vi "IMU Read.vi"(6 "Configuration":T2={"Accelerometer Bias"={"X (m/s)"=0.0, "Y (m/s)"=0.0, "Z (m/s)"=0.0}, "Gyroscope Bias"={"X (m/s)"=0.0, "Y (m/s)"=0.0, "Z (m/s)"=0.0}, "Steering Motor Gear Ratio"=0.0, "Steering Pully Gear Ratio"=0.0, "Steering Encoder CPR"=0.0, "Steering Motor Max RPM"=4000.0, "Wheelbase (m)"=1.12, "Fork Angle (rad)"=1.3, "Balancing Controller"={"Kp (/s)"=0.0, "Kd (1)"=0.0}, "Max Allowed Steering Angle (rad)"=0.7, "Task Periods"={"Emergency Stop (us)"=0, "IMU (us)"=0, "Steering Motor Encoder (us)"=0, "State Estimator (us)"=0, "Balancing Controller (us)"=0, "GNSS (us)"=0, "Logging (us)"=0, "Drive Motor (us)"=0, "Visualization (us)"=50000}, "Drive Motor Gear Ratio"=0.7, "lr"=0.0, "lf"=0.0, "lambda"=0.0, "k1"=0.0, "k2"=0.0, "e1_max"=0.0, "Ad_t"=0.0, "Bd_t"=0.0, "C_t"=0.0, "D_t"=0.0, "Wheel radius"=0.311}, 8 "Measurement In":refnum<data-value>, 9 "Flag IMU":dbl, 10 "IMU Handle":T3={"I2C address"=107}, 11 "Error In":errorcluster) -> (0 "Measurement Out":refnum<data-value>, 1 "IMU Data":T1, 3 "Error Out":errorcluster)   [LabVIEW 2021]
uses:
  IMU Handle.ctl
  Configuration/Configuration.ctl
  IMU Data.ctl
  State Estimator/Measurements.ctl
  Steering Motor Encoder/Steering Motor Encoder Data.ctl
  GNSS/GNSS Data.ctl
  <vilib>/myRIO/Instrument Drivers/Onboard IO/I2C/typedefs/I2C User Configuration.ctl
  <vilib>/myRIO/Instrument Drivers/Onboard IO/I2C/typedefs/I2C Transfer Rate.ctl
  <vilib>/myRIO/Instrument Drivers/Onboard IO/I2C/typedefs/I2C Reference.ctl
  <vilib>/myRIO/Common/Instrument Driver Framework/Utilities/typedefs/myRIO Generic Hardware Reference.ctl
  <vilib>/myRIO/Common/Instrument Driver Framework/Utilities/typedefs/Hardware Version Enum.ctl
  <vilib>/myRIO/Common/Instrument Driver Framework/Utilities/typedefs/myRIO v1.0 Reference.ctl
  <vilib>/myRIO/Common/Instrument Driver Framework/Utilities/typedefs/Generic FPGA Reference.ctl
  <vilib>/myRIO/Common/Instrument Driver Framework/myRIO v1.0/I2C/typedefs/I2C Channels Enum.ctl
  <vilib>/myRIO/Instrument Drivers/Onboard IO/I2C/typedefs/I2C Configuration.ctl
  <vilib>/userDefined/High Color/nirio_resource_hc.ctl
  <vilib>/myRIO/Common/Instrument Driver Framework/Utilities/vis/Is FPGA Ref Available.vi
  <vilib>/myRIO/Common/Instrument Driver Framework/myRIO v1.0/I2C/vis/myRIO v1.1 Open I2C.vi
  <vilib>/myRIO/Instrument Drivers/Onboard IO/I2C/vis/Configure.vi
  <vilib>/myRIO/Instrument Drivers/Onboard IO/I2C/vis/Write Read.vi
  <vilib>/myRIO/Common/Instrument Driver Framework/Utilities/vis/Validate Channels.vi
  <vilib>/myRIO/Common/Instrument Driver Framework/myRIO v1.0/I2C/vis/myRIO v1.0 Reserve I2C.vi
  <vilib>/myRIO/Common/Instrument Driver Framework/myRIO v1.0/I2C/vis/myRIO v1.0 Build MUX Configuration I2C.vi
  <vilib>/myRIO/Common/Instrument Driver Framework/myRIO v1.0/Resource Manager/vis/myRIO v1.0 Reserve Channel List.vi
  <vilib>/myRIO/Common/Instrument Driver Framework/myRIO v1.0/Resource Manager/vis/myRIO v1.0 Create Configuration List.vi
  <vilib>/myRIO/Common/Instrument Driver Framework/myRIO v1.0/Resource Manager/vis/myRIO v1.0 Reserve Channel.vi
  <vilib>/myRIO/Common/Instrument Driver Framework/myRIO v1.0/Resource Manager/vis/myRIO v1.0 Unreserve Channel.vi
  <vilib>/myRIO/Common/Instrument Driver Framework/myRIO v1.0/Resource Manager/vis/myRIO v1.0 Build Mutex Name.vi
  <vilib>/Utility/VariantDataType/GetNumericInfo.vi
  <vilib>/Utility/error.llb/Error Cluster From Error Code.vi
  <vilib>/myRIO/Common/Instrument Driver Framework/myRIO v1.0/myRIO v1.1 Open.vi
  <vilib>/myRIO/Common/Instrument Driver Framework/Utilities/vis/IO Manager.vi
  <vilib>/myRIO/Common/Instrument Driver Framework/Utilities/vis/Configuration Manager.vi
  <vilib>/myRIO/Common/Instrument Driver Framework/myRIO v1.0/Resource Manager/vis/myRIO v1.0 Configure IO.vi
  <vilib>/myRIO/Common/Instrument Driver Framework/myRIO v1.0/myRIO v1.0 Close.vi
  <vilib>/myRIO/Common/Instrument Driver Framework/myRIO v1.0/I2C/vis/myRIO v1.0 Configure I2C.vi
  <vilib>/myRIO/Common/Instrument Driver Framework/myRIO v1.0/I2C/vis/myRIO v1.0 Write I2C.vi
  <vilib>/myRIO/Common/Instrument Driver Framework/myRIO v1.0/I2C/vis/myRIO v1.0 Read I2C.vi
  <vilib>/myRIO/Express VI/Onboard IO/I2C/I2C Express VI.xnode
  <vilib>/myRIO/Instrument Drivers/Onboard IO/I2C/vis/myRIO I2C Open.xnode
  <vilib>/myRIO/Instrument Drivers/Onboard IO/I2C/I2C.lvlib
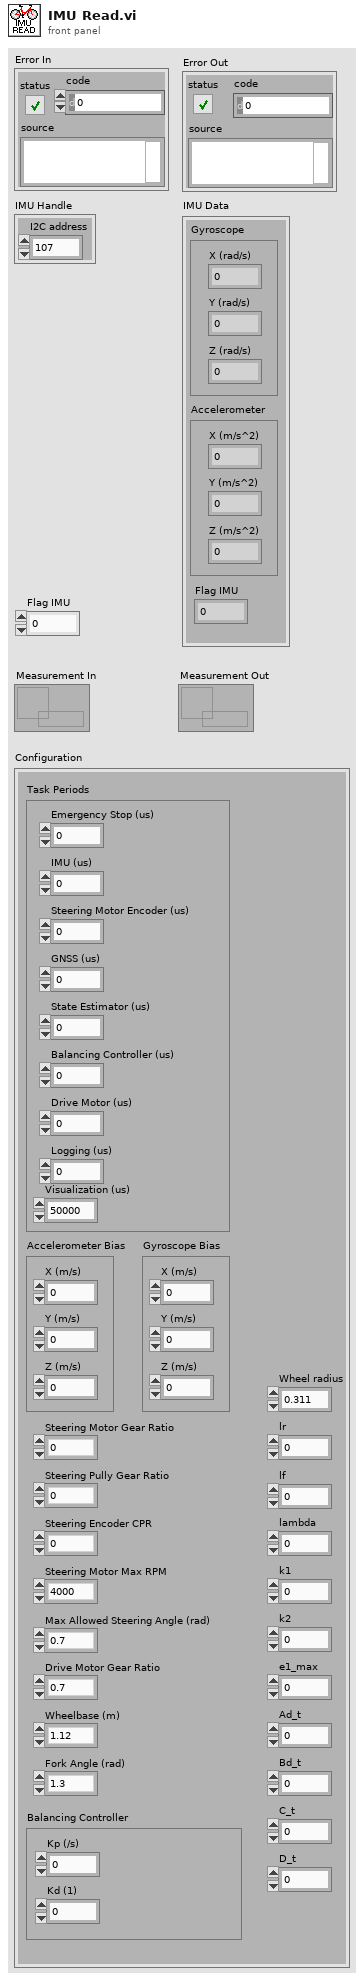
[diagram p1: front panel]
types:
  T1 = typedef "IMU Data.ctl" = cluster{"Gyroscope":cluster{"X (rad/s)":dbl, "Y (rad/s)":dbl, "Z (rad/s)":dbl}, "Accelerometer":cluster{"X (m/s^2)":dbl, "Y (m/s^2)":dbl, "Z (m/s^2)":dbl}, "Flag IMU":dbl}
  T2 = typedef "Configuration.ctl" = cluster{"Accelerometer Bias":cluster{"X (m/s)":dbl, "Y (m/s)":dbl, "Z (m/s)":dbl}, "Gyroscope Bias":cluster{"X (m/s)":dbl, "Y (m/s)":dbl, "Z (m/s)":dbl}, "Steering Motor Gear Ratio":dbl, "Steering Pully Gear Ratio":dbl, "Steering Encoder CPR":dbl, "Steering Motor Max RPM":dbl, "Wheelbase (m)":dbl, "Fork Angle (rad)":dbl, "Balancing Controller":cluster{"Kp (/s)":dbl, "Kd (1)":dbl}, "Max Allowed Steering Angle (rad)":dbl, "Task Periods":cluster{"Emergency Stop (us)":i64, "IMU (us)":i64, "Steering Motor Encoder (us)":i64, "State Estimator (us)":i64, "Balancing Controller (us)":i64, "GNSS (us)":i64, "Logging (us)":i64, "Drive Motor (us)":i64, "Visualization (us)":i64}, "Drive Motor Gear Ratio":dbl, "lr":dbl, "lf":dbl, "lambda":dbl, "k1":dbl, "k2":dbl, "e1_max":dbl, "Ad_t":dbl, "Bd_t":dbl, "C_t":dbl, "D_t":dbl, "Wheel radius":dbl}
  T3 = typedef "IMU Handle.ctl" = cluster{"I2C address":u8}
  T4 = cluster{"X (m/s)":dbl, "Y (m/s)":dbl, "Z (m/s)":dbl}
  T5 = cluster{cluster{dbl, dbl, dbl}, cluster{dbl, dbl, dbl}, "Flag IMU":dbl}
  T6 = typedef "Measurements.ctl" = cluster{"IMU Data":T1, "Steering Motor Encoder Data":T7, "GNSS Data":T8}
  T7 = typedef "Steering Motor Encoder Data.ctl" = cluster{"Encoder Position (counts)":i32, "Steering Angle (rad)":dbl, "Flag Steering Encoder":dbl}
  T8 = typedef "GNSS Data.ctl" = cluster{"Latitude (rad)":dbl, "Longitude (rad)":dbl, "Altitude (m)":dbl, "Speed (m/s)":dbl, "Heading (rad)":dbl, "Fix Quality":i32, "Number of Satellites":i32, "Latitude (deg)":dbl, "Longitude (deg)":dbl, "Flag GNSS":dbl}
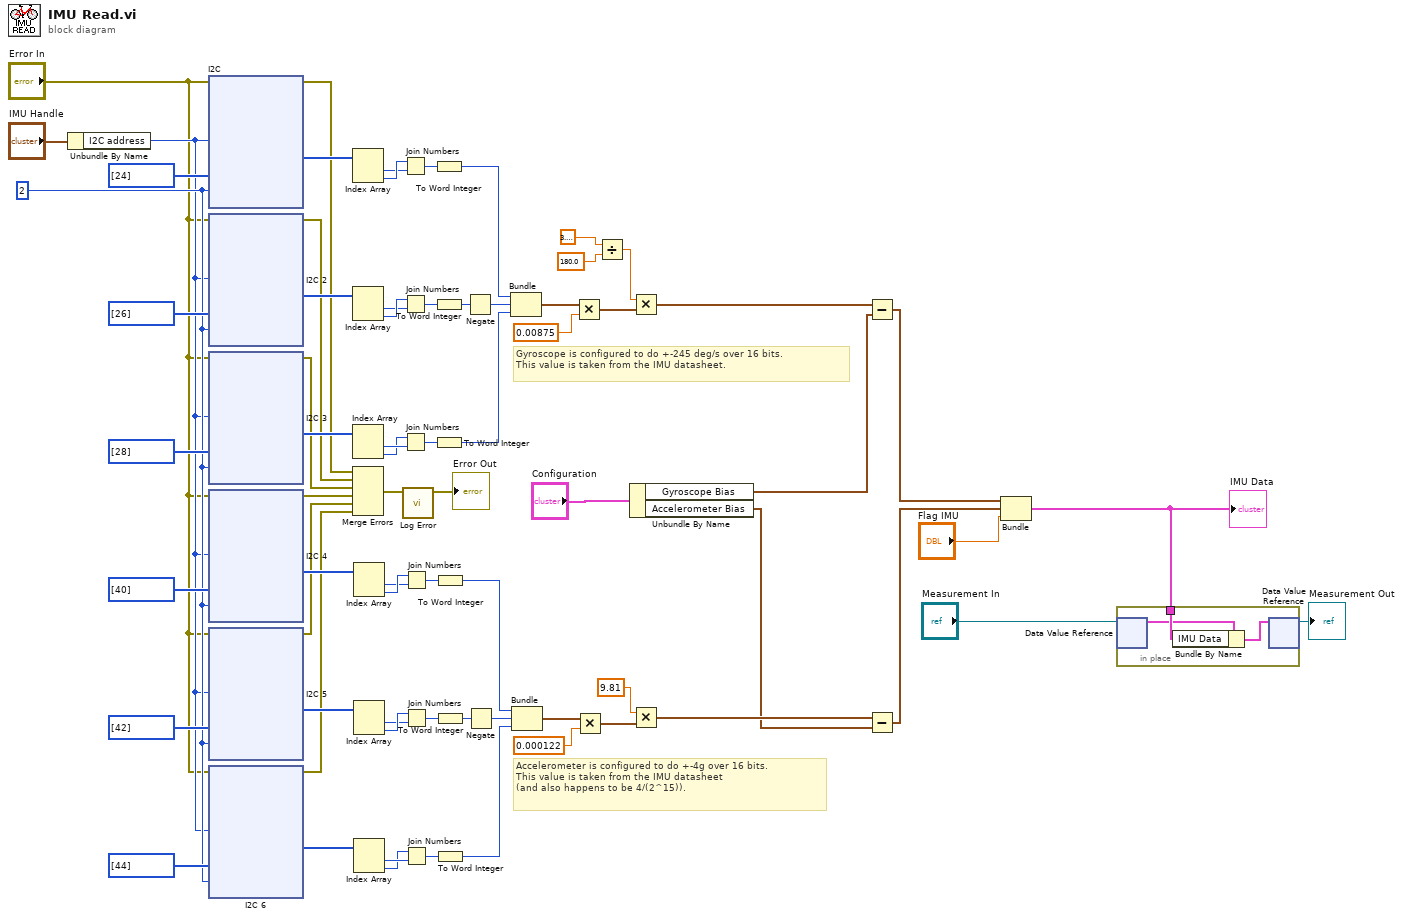
[diagram p0: block diagram]
diagram:
  w65 = u32 2 ("Byte Count")
  # "Accelerometer is configured to do +-4g over 16 bits.\nThis value is taken from the IMU datasheet\n(and also happens to be 4/(2^15))."
  # "Gyroscope is configured to do +-245 deg/s over 16 bits.\nThis value is taken from the IMU datasheet."
  n1 = Unbundle By Name("IMU Handle") -> ("I2C address"=w64:u8)
  n2 = xnode "I2C"("Slave Address (7-bit)"=w64, "Bytes to Write"=u8[] [24], "Byte Count"=w65, "error in (no error)"="Error In") -> ("Bytes Read"=w47:u8[], "error out"=w18:errorcluster)
  n3 = xnode "I2C 2"("Slave Address (7-bit)"=w64, "Bytes to Write"=u8[] [26], "Byte Count"=w65, "error in (no error)"="Error In") -> ("Bytes Read"=w46:u8[], "error out"=w17:errorcluster)
  n4 = xnode "I2C 3"("Slave Address (7-bit)"=w64, "Bytes to Write"=u8[] [28], "Byte Count"=w65, "error in (no error)"="Error In") -> ("Bytes Read"=w45:u8[], "error out"=w16:errorcluster)
  n5 = xnode "I2C 4"("Slave Address (7-bit)"=w64, "Bytes to Write"=u8[] [40], "Byte Count"=w65, "error in (no error)"="Error In") -> ("Bytes Read"=w35:u8[], "error out"=w19:errorcluster)
  n6 = xnode "I2C 5"("Slave Address (7-bit)"=w64, "Bytes to Write"=u8[] [42], "Byte Count"=w65, "error in (no error)"="Error In") -> ("Bytes Read"=w34:u8[], "error out"=w14:errorcluster)
  n7 = xnode "I2C 6"("Slave Address (7-bit)"=w64, "Bytes to Write"=u8[] [44], "Byte Count"=w65, "error in (no error)"="Error In") -> ("Bytes Read"=w33:u8[], "error out"=w15:errorcluster)
  n8 = Index Array(array=w47) -> (element #1=w59:u8, element #2=w60:u8)  [unwired: 2 in]
  n9 = Index Array(array=w46) -> (element #1=w61:u8, element #2=w62:u8)  [unwired: 2 in]
  n10 = Index Array(array=w45) -> (element #1=w55:u8, element #2=w54:u8)  [unwired: 2 in]
  n11 = Merge Errors(w18, w17, w16, w19, w14, w15) -> (w4:errorcluster)
  n12 = Index Array(array=w35) -> (element #1=w41:u8, element #2=w42:u8)  [unwired: 2 in]
  n13 = Index Array(array=w34) -> (element #1=w43:u8, element #2=w44:u8)  [unwired: 2 in]
  n14 = Index Array(array=w33) -> (element #1=w37:u8, element #2=w36:u8)  [unwired: 2 in]
  n15 = Join Numbers(hi=w60, lo=w59) -> ((hi.lo)=w56:u16)
  n16 = Join Numbers(hi=w62, lo=w61) -> ((hi.lo)=w57:u16)
  n17 = Join Numbers(hi=w54, lo=w55) -> ((hi.lo)=w58:u16)
  n18 = Join Numbers(hi=w42, lo=w41) -> ((hi.lo)=w38:u16)
  n19 = Join Numbers(hi=w44, lo=w43) -> ((hi.lo)=w39:u16)
  n20 = Join Numbers(hi=w36, lo=w37) -> ((hi.lo)=w40:u16)
  n21 = call "Log Error.vi"("Error In"=w4) -> ("Error Out"=→"Error Out":errorcluster)  [unwired: 10 in]
  n22 = To Word Integer(number=w56) -> (16bit integer=w53:i16)
  n23 = To Word Integer(number=w57) -> (16bit integer=w51:i16)
  n24 = To Word Integer(number=w58) -> (16bit integer=w52:i16)
  n25 = To Word Integer(number=w38) -> (16bit integer=w31:i16)
  n26 = To Word Integer(number=w39) -> (16bit integer=w30:i16)
  n27 = To Word Integer(number=w40) -> (16bit integer=w29:i16)
  n28 = Negate(x=w51) -> (-x=w50:i16)
  n29 = Negate(x=w30) -> (-x=w32:i16)
  n30 = Bundle "Bundle"(w53, w50, w52) -> (w49:cluster{i16, i16, i16})  [unwired: 1 in]
  n31 = Bundle "Bundle"(w31, w32, w29) -> (w25:cluster{i16, i16, i16})  [unwired: 1 in]
  n32 = Multiply(x=w49, y=0.00875) -> (x*y=w24:cluster{dbl, dbl, dbl})
  n33 = Multiply(x=w25, y=0.000122) -> (x*y=w28:cluster{dbl, dbl, dbl})
  n34 = Divide(x=3.141592653589793, y=180.0) -> (x/y=w23:dbl)
  n35 = Unbundle By Name("Configuration") -> ("Gyroscope Bias"=w13:T4, "Accelerometer Bias"=w1:T4)
  n36 = Multiply(x=w23, y=w24) -> (x*y=w20:cluster{dbl, dbl, dbl})
  n37 = Multiply(x=9.81 ("y"), y=w28) -> (x*y=w12:cluster{dbl, dbl, dbl})
  n38 = Subtract(x=w20, y=w13) -> (x-y=w11:cluster{dbl, dbl, dbl})
  n39 = Subtract(x=w12, y=w1) -> (x-y=w10:cluster{dbl, dbl, dbl})
  n40 = Bundle(w11, w10, "Flag IMU"="Flag IMU") -> (w2:T5)  [unwired: 1 in]
  "IMU Data" <- w2
  n41 = in-place {
    in-place-border: w2 -> [w73]
    n42 = in-place-dvr #1("Measurement In") -> (w72:T6)  [unwired: 1 out]
    n43 = Bundle By Name(cluster=w72, "IMU Data"=w73) -> (w74:T6)
    n44 = in-place-dvr #1(w74) -> (→"Measurement Out":refnum<data-value>)  [unwired: 1 out]
  }
